vi "Initialize AI Task.vi"(8 "error in (no error)":errorcluster, 11 "BNT_ULx-MCSV-AIAvg in":refnum<class "BNT_ULx-MCSV-AIAvg.lvclass">) -> (0 "error out":errorcluster, 3 "AI ULx Task":refnum<k24>)   [LabVIEW 2021, in "BNT_ULx.lvlib" / "BNT_ULx-MCSV-AIAvg.lvclass"]
doc: "Initialize DAQmx Analog Input task.\n\n<b>Default Implementation:</b> Analog Input Voltage\n\nThis dynamic dispatch VI can be overritten by derived classes to implement other analog input tasks."
uses:
  BNT_ULx-MCSV-AIAvg.lvclass
  <vilib>/ULx/ULx_LV.dll
  BNT_ULx-MCSV-AIAvg.lvclass/BNT_ULx-MCSV-AIAvg.ctl
  <vilib>/ULx/Timing.llb/ULx Timing (Sample Clock).vi
  BNT_ULx-MCSV/BNT_ULx-MCSV.lvclass
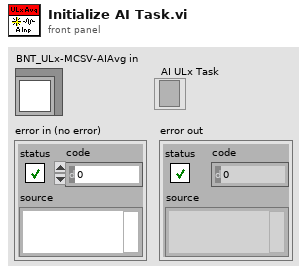
[diagram p1: front panel]
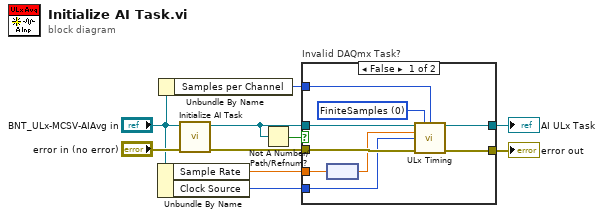
[diagram p0: block diagram]
diagram:
  n1 = Unbundle By Name("BNT_ULx-MCSV-AIAvg in") -> ("Sample Rate"=w7:dbl[unit], "Clock Source"=w6:i32)
  n2 = Unbundle By Name("BNT_ULx-MCSV-AIAvg in") -> ("Samples per Channel"=w10:i32)
  n3 = call-parent "Initialize AI Task.vi"("error in (no error)"="error in (no error)", "BNT_ULx-MCSV in"="BNT_ULx-MCSV-AIAvg in") -> ("error out"=w3:errorcluster, "AI ULx Task"=w1:refnum<k24>)  [unwired: 8 in]
  n4 = Not A Number/Path/Refnum?(number/path/refnum=w1) -> (NaN/Path/Refnum?=w2:bool)
  n5 = case "Invalid DAQmx Task?" shown="False" w2 {
    tunnel: w10 -> [w14 _]
    tunnel: w7 -> [w19 _]
    tunnel: w6 -> [w12 _]
    tunnel: [w11 w21] -> w5
    tunnel: [w17 w20] -> w4
    tunnel: w1 -> [w15 w21]
    tunnel: w3 -> [w16 w20]
    frame False {
      w18 = 0 items=["FiniteSamples", "ContinuousSamples"] ("sample mode")
      n6 = node(w19) -> (w13:dbl)
      n7 = call-poly <vilib>:"ULx Timing.vi"("task in"=w15, "sample mode"=w18, "samples per channel"=w14, "rate"=w13, "clock source"=w12, "error in"=w16) -> ("task out"=w11:refnum<k24>, "error out"=w17:errorcluster)  [unwired: 8 in]
    }
    frame True {
    }
  }
  "error out" <- w4
  "AI ULx Task" <- w5
